vi "Close.vi"(8 "error in":errorcluster, 11 "NetworkHandler in":refnum<class "StreamLogHandle.lvclass">) -> (0 "error out":errorcluster)   [LabVIEW 2024, in "StreamLogHandle.lvclass"]
doc: "Closes the log-file. This method should be called when the ``Logger`` gets closed or the handler is removed from the ``Logger``.\n\n____\nHAMPEL SOFTWARE ENGINEERING v2.2.2 (2025-01-16 15:41)"
uses:
  StreamLogHandle.lvclass
  StreamLogHandle.lvclass/StreamLogHandle.ctl
  Stream/IStreamWriter/IStreamWriter.lvclass
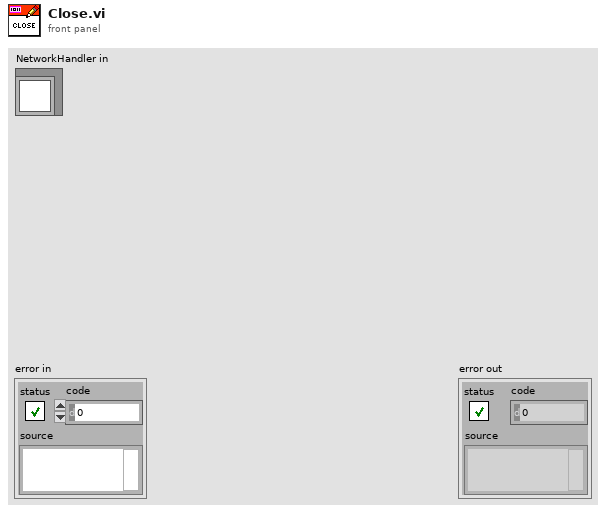
[diagram p1: front panel]
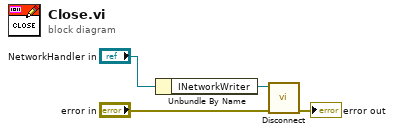
[diagram p0: block diagram]
diagram:
  n1 = Unbundle By Name("NetworkHandler in") -> ("INetworkWriter"=w3:refnum<class "IStreamWriter.lvclass">)
  n2 = call-dynamic "Disconnect.vi"("error in (no error)"="error in", "INetworkWriter in"=w3) -> ("error out"=→"error out":errorcluster)  [unwired: 8 in, 1 out]
